vi "4.vi"() -> ()   [LabVIEW 2019]
uses:
  <vilib>/imath/engines/lvmath/Plug In/_Char/NIMS_CH_character datatype.ctl
  <vilib>/imath/engines/lvmath2/RunTimeEngine/Managers/WorkSpace/UID Generator.vi
  <vilib>/imath/engines/lvmath/Plug In/_Char/NIMS_CH_Character RV to String.vi
  <vilib>/imath/engines/lvmath2/RunTimeEngine/BuiltInFunctions/wavread/NIMS_wavread(Str,I32V).vi
  <vilib>/imath/engines/lvmath2/RunTimeEngine/BuiltInFunctions/length/NIMS_length(GM).vi
  <instcachedir>/0/NIMS_length(GM)_47CEC356FCE0482D9BA47DC61C99F2C7.lvgen/NIMS_length(GM)_47CEC356FCE0482D9BA47DC61C99F2C7_000.vi
  <vilib>/imath/engines/lvmath2/RunTimeEngine/BuiltInFunctions/size/NIMS_I32Row=size(GM).vi
  <instcachedir>/0/NIMS_I32Row=size(GM)_10ACDCB9F1F84A7E9F42C91D87611FB5.lvgen/NIMS_I32Row=size(GM)_10ACDCB9F1F84A7E9F42C91D87611FB5_001.vi
  <vilib>/imath/engines/lvmath2/RunTimeEngine/BuiltInFunctions/randnormal/NIMS_randnormal(I32V).vi
  <vilib>/imath/engines/lvmath2/RunTimeEngine/ErrorHandling/NIMS_Create Error From Enums.vi
  <vilib>/imath/engines/lvmath2/RunTimeEngine/BuiltInFunctions/mean/NIMS_RRow=mean(RM,I32).vi
  <vilib>/imath/engines/lvmath2/RunTimeEngine/ArithmeticOperatorToken/NIMS_ArithmeticOperator_minus.vi
  <instcachedir>/0/NIMS_ArithmeticOperator_minus_12BFF9710EA5430A9EE87C5BC3F65186.lvgen/NIMS_ArithmeticOperator_minus_12BFF9710EA5430A9EE87C5BC3F65186_002.vi
  <vilib>/imathl/engines/lvmath/Functions/Error Handling/Create Error.vi
  <vilib>/imath/engines/lvmath2/RunTimeEngine/ArithmeticOperatorToken/NIMS_ArithmeticOperator_times.vi
  <instcachedir>/0/NIMS_ArithmeticOperator_times_B08792E9E3A74C8190DF4DEBB44E818C.lvgen/NIMS_ArithmeticOperator_times_B08792E9E3A74C8190DF4DEBB44E818C_007.vi
  <vilib>/imath/engines/lvmath2/RunTimeEngine/BuiltInFunctions/sum/NIMS_sum(GM,Sca).vi
  <instcachedir>/0/NIMS_sum(GM,Sca)_5A881C89F56546CCB4EF2C2326C78C27.lvgen/NIMS_sum(GM,Sca)_5A881C89F56546CCB4EF2C2326C78C27_001.vi
  <vilib>/imath/engines/lvmath2/RunTimeEngine/BuiltInFunctions/std/NIMS_std(GM,RV).vi
  <instcachedir>/0/NIMS_std(GM,RV)_457C706E3C994DBC8BC829DDC02A99D1.lvgen/NIMS_std(GM,RV)_457C706E3C994DBC8BC829DDC02A99D1_001.vi
  <vilib>/imath/engines/lvmath2/RunTimeEngine/ArithmeticOperatorToken/NIMS_ArithmeticOperator_rightdivmx(C,C).vi
  <instcachedir>/0/NIMS_ArithmeticOperator_rightdivmx(C,C)_4C9834AF73264B85B2EC0ABB36B07CCF.lvgen/NIMS_ArithmeticOperator_rightdivmx(C,C)_4C9834AF73264B85B2EC0ABB36B07CCF_000.vi
  <vilib>/imath/engines/lvmath2/RunTimeEngine/ArithmeticOperatorToken/NIMS_ArithmeticOperator_multmx.vi
  <instcachedir>/0/NIMS_ArithmeticOperator_multmx_77F1D2D6F4D94BA7A97C4E7185C02392.lvgen/NIMS_ArithmeticOperator_multmx_77F1D2D6F4D94BA7A97C4E7185C02392_006.vi
  <vilib>/imath/engines/lvmath2/RunTimeEngine/ArithmeticOperatorToken/NIMS_ArithmeticOperator_plus.vi
  <instcachedir>/0/NIMS_ArithmeticOperator_plus_5C9385B0197D46E2B844C41E02F9EC39.lvgen/NIMS_ArithmeticOperator_plus_5C9385B0197D46E2B844C41E02F9EC39_010.vi
  C:/Users/13087/Documents/LabVIEW Data/MathScriptVIs/MCStatic_41946317732_ffc3f065e415bbdbbc756a963756b0a5.vi
  <instcachedir>/0/MCStatic_41946317732_ffc3f065e415bbdbbc756a963756b0a5_3C9C68647ABA497AB3A212223C11C42A.lvgen/MCStatic_41946317732_ffc3f065e415bbdbbc756a963756b0a5_3C9C68647ABA497AB3A212223C11C42A_000.vi
  <vilib>/imath/engines/lvmath2/RunTimeEngine/UserFunctionToken/NIMS_UserFunction_CondDefined.vi
  <instcachedir>/0/NIMS_UserFunction_CondDefined_34DB21F43CC6438AB39490E17DD0B947.lvgen/NIMS_UserFunction_CondDefined_34DB21F43CC6438AB39490E17DD0B947_000.vi
  <vilib>/imath/engines/lvmath2/RunTimeEngine/MatrixToken/NIMS_MatrixToken_RV_RV.vi
  <instcachedir>/0/NIMS_MatrixToken_RV_RV_226199DAD5A543BDA46C6E2C67E5DD1B.lvgen/NIMS_MatrixToken_RV_RV_226199DAD5A543BDA46C6E2C67E5DD1B_002.vi
  <vilib>/imath/engines/lvmath2/RunTimeEngine/MatrixToken/NIMS_MatrixToken_M_RV.vi
  <instcachedir>/0/NIMS_MatrixToken_M_RV_2CF9F93F920A4B3FA1DA30AAEAA659ED.lvgen/NIMS_MatrixToken_M_RV_2CF9F93F920A4B3FA1DA30AAEAA659ED_001.vi
  <vilib>/imath/engines/lvmath/Functions/Error Handling/MergeErrorsWrapper.vi
  C:/Users/13087/Documents/LabVIEW Data/MathScriptVIs/MCStatic_41946317732_d4f867800144aa32764446d58d9fe4fa.vi
  <instcachedir>/0/MCStatic_41946317732_d4f867800144aa32764446d58d9fe4fa_91776CB147E44557B1508EEF89087DE1.lvgen/MCStatic_41946317732_d4f867800144aa32764446d58d9fe4fa_91776CB147E44557B1508EEF89087DE1_000.vi
  <vilib>/imath/engines/lvmath2/RunTimeEngine/RangeToken/NIMS_Range_R2 - Integer.vi
  <instcachedir>/0/NIMS_Range_R2 - Integer_8A7AF97FD8504F909FC0FDE0F1D1FB54.lvgen/NIMS_Range_R2 - Integer_8A7AF97FD8504F909FC0FDE0F1D1FB54_000.vi
  <vilib>/imath/engines/lvmath2/RunTimeEngine/CommandStatement/MC_CommandStatement_break.vi
  <vilib>/imath/engines/lvmath2/RunTimeEngine/IndexRead/NIMS M(S,S).vi
  <instcachedir>/0/NIMS M(S,S)_AC51E74150A542F7991B9634C66F3096.lvgen/NIMS M(S,S)_AC51E74150A542F7991B9634C66F3096_002.vi
  <vilib>/imath/engines/lvmath2/RunTimeEngine/IndexRead/NIMS M(R2,$).vi
  <instcachedir>/0/NIMS M(R2,$)_AD8DC2FC79024024B2717E13B4A0EB4B.lvgen/NIMS M(R2,$)_AD8DC2FC79024024B2717E13B4A0EB4B_001.vi
  <vilib>/imath/engines/lvmath2/RunTimeEngine/VariableToken/NIMS_VariableToken_CondDefinedDefinedByReplace.vi
  <instcachedir>/0/NIMS_VariableToken_CondDefinedDefinedByReplace_D162CFFC24174562A9FEA619A91E1A56.lvgen/NIMS_VariableToken_CondDefinedDefinedByReplace_D162CFFC24174562A9FEA619A91E1A56_000.vi
  <vilib>/imath/engines/lvmath2/RunTimeEngine/IndexReplace/NIMS V(R2)=M.vi
  <instcachedir>/0/NIMS V(R2)=M_BE8307057F984B3BBBCBCED1D5C0FCE7.lvgen/NIMS V(R2)=M_BE8307057F984B3BBBCBCED1D5C0FCE7_000.vi
  <vilib>/imath/engines/lvmath2/RunTimeEngine/IndexRead/NIMS M(S,$).vi
  <instcachedir>/0/NIMS M(S,$)_F24F360562DE41D8BE234322A2E15C65.lvgen/NIMS M(S,$)_F24F360562DE41D8BE234322A2E15C65_000.vi
  <instcachedir>/0/NIMS_length(GM)_47CEC356FCE0482D9BA47DC61C99F2C7.lvgen/NIMS_length(GM)_47CEC356FCE0482D9BA47DC61C99F2C7_005.vi
  <vilib>/imath/engines/lvmath2/RunTimeEngine/BuiltInFunctions/length/NIMS_length(GV).vi
  <instcachedir>/0/NIMS_length(GV)_08A3D13377FD4E4B96F5795FBF3698FA.lvgen/NIMS_length(GV)_08A3D13377FD4E4B96F5795FBF3698FA_000.vi
  <vilib>/imath/engines/lvmath2/RunTimeEngine/BuiltInFunctions/zeros/NIMS_V=zeros(I32,I32).vi
  <vilib>/imath/engines/lvmath2/RunTimeEngine/BuiltInFunctions/crosscorr/NIMS_crosscorr(GM,GM,Str).vi
  <instcachedir>/0/NIMS_crosscorr(GM,GM,Str)_E2B688A058B24E62B61F0BB8631EA9D6.lvgen/NIMS_crosscorr(GM,GM,Str)_E2B688A058B24E62B61F0BB8631EA9D6_001.vi
  <vilib>/imath/engines/lvmath2/RunTimeEngine/IndexReplace/NIMS M(S,S)=S.vi
  <instcachedir>/0/NIMS M(S,S)=S_F60428D0350A4667AE68E0C0372F4DD1.lvgen/NIMS M(S,S)=S_F60428D0350A4667AE68E0C0372F4DD1_001.vi
  <vilib>/imath/engines/lvmath2/RunTimeEngine/BuiltInFunctions/max/1 input/NIMS_max(CM).vi
  <instcachedir>/0/NIMS_max(CM)_ECFF9CEF2CF74B92B05BC258ECD38873.lvgen/NIMS_max(CM)_ECFF9CEF2CF74B92B05BC258ECD38873_000.vi
  <vilib>/imath/engines/lvmath2/RunTimeEngine/IndexReplace/NIMS M(S,S)=V.vi
  <instcachedir>/0/NIMS M(S,S)=V_D2B0CC22DFC34594AC148C08E45838CE.lvgen/NIMS M(S,S)=V_D2B0CC22DFC34594AC148C08E45838CE_000.vi
  <instcachedir>/0/NIMS M(S,$)_F24F360562DE41D8BE234322A2E15C65.lvgen/NIMS M(S,$)_F24F360562DE41D8BE234322A2E15C65_001.vi
  <vilib>/imath/engines/lvmath2/RunTimeEngine/BuiltInFunctions/max/1 input/NIMS_max(CV).vi
  <instcachedir>/0/NIMS_max(CV)_590AF7B4F5274293AE83668956F92BC1.lvgen/NIMS_max(CV)_590AF7B4F5274293AE83668956F92BC1_000.vi
  <vilib>/imath/engines/lvmath2/RunTimeEngine/RowToken/NIMS_RowToken_M_SorRV.vi
  <instcachedir>/0/NIMS_RowToken_M_SorRV_8B225983F7C241309B26ACF9CFA182E8.lvgen/NIMS_RowToken_M_SorRV_8B225983F7C241309B26ACF9CFA182E8_001.vi
  <vilib>/imath/engines/lvmath2/RunTimeEngine/BuiltInFunctions/mx_to_str/NIMS_mx_to_str(RM,CS).vi
  <vilib>/imath/engines/lvmath/Plug In/_Char/NIMS_CH_String to Character Array.vi
  <vilib>/imath/engines/lvmath2/RunTimeEngine/ErrorHandling/NIMS_Error From Error Code.vi
  <vilib>/imath/engines/lvmath2/RunTimeEngine/IndexRead/NIMS V(R2).vi
  <instcachedir>/0/NIMS V(R2)_C76619605A0E4E9F8B2FA9389712AC47.lvgen/NIMS V(R2)_C76619605A0E4E9F8B2FA9389712AC47_002.vi
  <vilib>/imath/engines/lvmath2/RunTimeEngine/BuiltInFunctions/strreplace/NIMS_strreplace.vi
  <vilib>/imath/engines/lvmath2/RunTimeEngine/VariableToken/NIMS_VariableToken_CondDefined.vi
  <instcachedir>/0/NIMS_VariableToken_CondDefined_30C3C94EAC01413DA882E848DEC89944.lvgen/NIMS_VariableToken_CondDefined_30C3C94EAC01413DA882E848DEC89944_000.vi
  <vilib>/imath/engines/lvmath2/RunTimeEngine/NodeEndStatement/NIMS_NodeEndStatement_Output.vi
  <instcachedir>/0/NIMS_NodeEndStatement_Output_53EC0D466D134D7ABD903AC30B43404B.lvgen/NIMS_NodeEndStatement_Output_53EC0D466D134D7ABD903AC30B43404B_008.vi
  <instcachedir>/0/NIMS_NodeEndStatement_Output_53EC0D466D134D7ABD903AC30B43404B.lvgen/NIMS_NodeEndStatement_Output_53EC0D466D134D7ABD903AC30B43404B_001.vi
  <instcachedir>/0/NIMS_NodeEndStatement_Output_53EC0D466D134D7ABD903AC30B43404B.lvgen/NIMS_NodeEndStatement_Output_53EC0D466D134D7ABD903AC30B43404B_000.vi
  <instcachedir>/0/NIMS_NodeEndStatement_Output_53EC0D466D134D7ABD903AC30B43404B.lvgen/NIMS_NodeEndStatement_Output_53EC0D466D134D7ABD903AC30B43404B_002.vi
  <instcachedir>/0/NIMS_NodeEndStatement_Output_53EC0D466D134D7ABD903AC30B43404B.lvgen/NIMS_NodeEndStatement_Output_53EC0D466D134D7ABD903AC30B43404B_003.vi
  <vilib>/imath/engines/lvmath2/RunTimeEngine/ErrorHandling/NIMS_Finalize Error.vi
  C:/Users/13087/Documents/LabVIEW Data/number_sig.m
  C:/Users/13087/Documents/LabVIEW Data/sigfilter.m
panel:
  out "去噪信号":dbl[](graph)
  out "噪声信号":dbl[][](graph)
  out "加噪声信号":dbl[][](graph)
  out "原始信号":dbl[][](graph)
  out "识别结果":string
  out "信号总时间":dbl
  out "信号采样频率":dbl
  in  "SNR":dbl=10.0
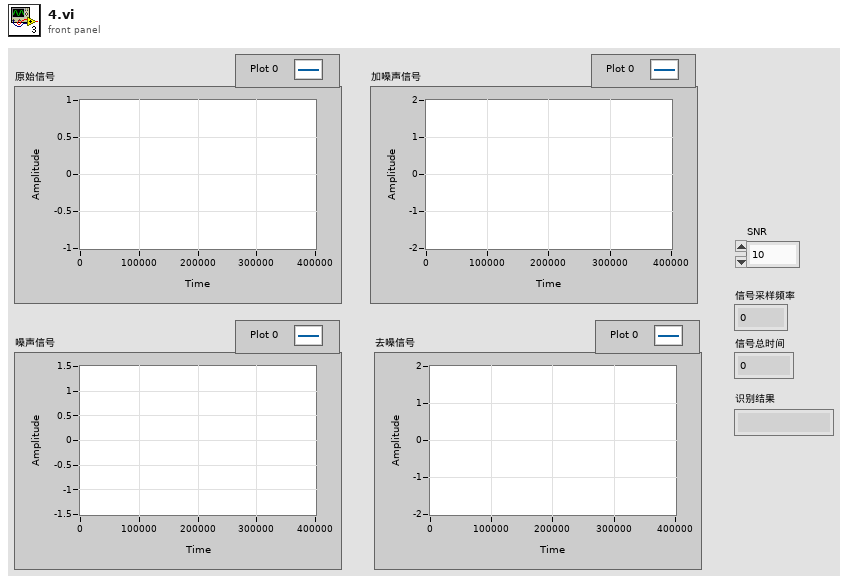
[diagram p1: front panel]
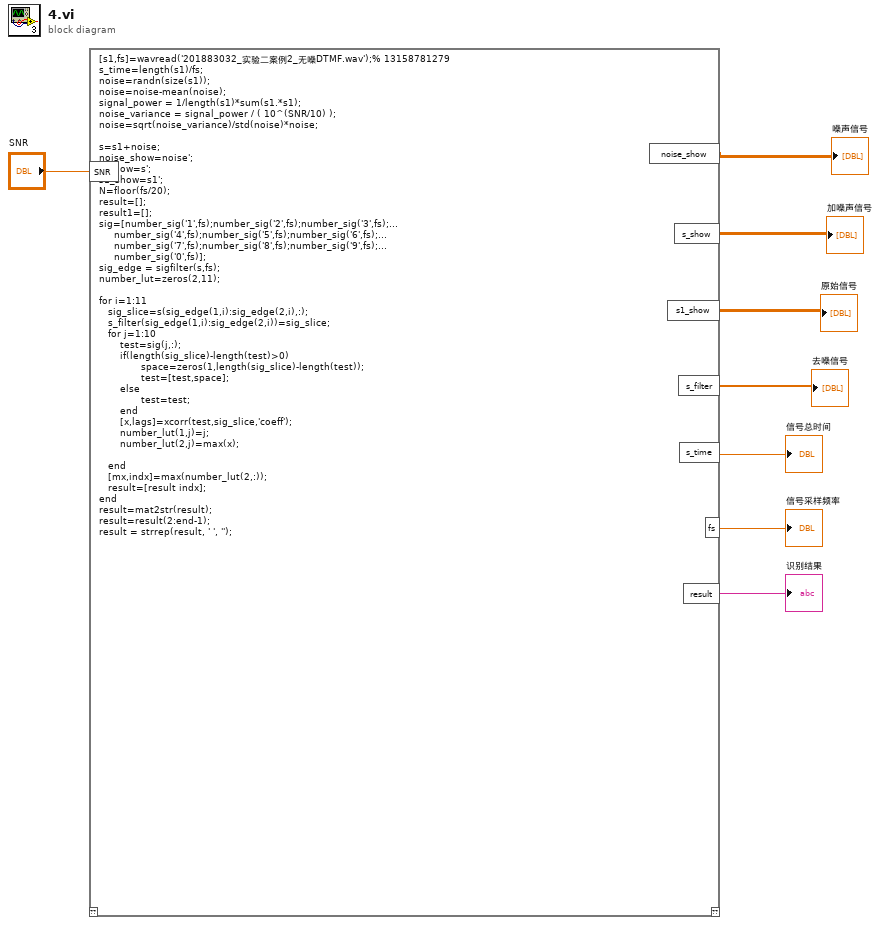
[diagram p0: block diagram]
diagram:
  n1 = mathscript code="[s1,fs]=wavread('201883032_实验二案例2_无噪DTMF.wav');% 13158781279\ns_time=length(s1)/fs;\nnoise=randn(size(s1));\nnoise=noise-mean(noise);\nsignal_power = 1/length(s1)*sum(s1.*s1);\nnoise_variance = signal_power / ( 10^(SNR/10) );\nnoise=sqrt(noise_variance)/std(noise)*noise;\n\ns=s1+noise;\nnoise_show=noise';\ns_show=s';\ns1_show=s1';\nN=floor(fs/20);\nresult=[];\nresult1=[];\nsig=[number_sig('1',fs);number_sig('2',fs);number_sig('3',fs);...\n     number_sig('4',fs);number_sig('5',fs);number_sig('6',fs);...\n     number_sig('7',fs);number_sig('8',fs);number_sig('9',fs);...\n     number_sig('0',fs)];\nsig_edge = sigfilter(s,fs);\nnumber_lut=zeros(2,11);\n\nfor i=1:11\n   sig_slice=s(sig_edge(1,i):sig_edge(2,i),:); \n   s_filter(sig_edge(1,i):sig_edge(2,i))=sig_slice;\n   for j=1:10\n       test=sig(j,:);\n       if(length(sig_slice)-length(test)>0)\n              space=zeros(1,length(sig_slice)-length(test));\n              test=[test,space];\n       else\n              test=test;\n       end\n       [x,lags]=xcorr(test,sig_slice,'coeff');\n       number_lut(1,j)=j;\n       number_lut(2,j)=max(x);\n\n   end\n   [mx,indx]=max(number_lut(2,:));\n   result=[result indx];\nend\nresult=mat2str(result);\nresult=result(2:end-1);\nresult = strrep(result, ' ', '');"("SNR"="SNR") -> ("noise_show"=→"噪声信号":cdb[][], "s_show"=→"加噪声信号":cdb[][], "s1_show"=→"原始信号":dbl[][], "s_filter"=→"去噪信号":cdb[], "s_time"=→"信号总时间":dbl, "fs"=→"信号采样频率":dbl, "result"=→"识别结果":string)  [unwired: 1 in, 1 out]
